vi "Fit Data.vi"(8 "error in":errorcluster, 10 "Data In":dbl[](array[numeric]), 11 "DFT-1 in":refnum<class "DFT-1.lvclass">) -> (0 "error out":errorcluster, 3 "DFT-1 out":refnum<class "DFT-1.lvclass">)   [LabVIEW 2014, in "Exponential Fit Library.lvlib" / "DFT-1.lvclass"]
doc: "Calculate tau from the first frequency component of the DFT using:\n\nbeta = 1/dt*ln(Re(F(k)/Im(F(k)*sin(w_k*dt) + cos(w_k*dt))\n\nwhere k = 1 and assuming unit spacing in time. Then, \n\ntau = 1/beta\n\nThe scale (A) and offset (B) are calculated as:\n\nA = (w^2+k^2)/ k*Re[F(n=1)]*dt/(1-exp(-k*tm)\nB = F(0)/N - A/(k*tm)*[1-exp(-k*tm)]\n\nwhere N is the number of samples, k = 1/tau, w = omega = 2*pi/tm, tm = N*dt, F(0) is the DC component of the FFT and Re[F(n=1)] is the real term of the first frequency component in the FFT spectrum. These computations are taken from Mazurenka et al. (2005) and are used in the determination of the uncertainty in the term tau (e_tau)."
uses:
  DFT-1.lvclass
  Fit Exponential.lvclass/Fit Exponential.ctl
  DFT-1.lvclass/DFT-1.ctl
  <vilib>/Analysis/2dsp.llb/Real FFT.vi
  Read Size.vi
  Read Sin.vi
  Read Cos.vi
  Read Dt.vi
  Write Output.vi
  Fit Exponential.lvclass
  <vilib>/Analysis/NI_AALPro.lvlib
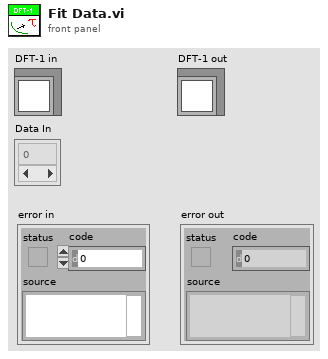
[diagram p1: front panel]
types:
  T1 = cluster{"A":dbl, "B":dbl, "tau":dbl, "e_tau":dbl}
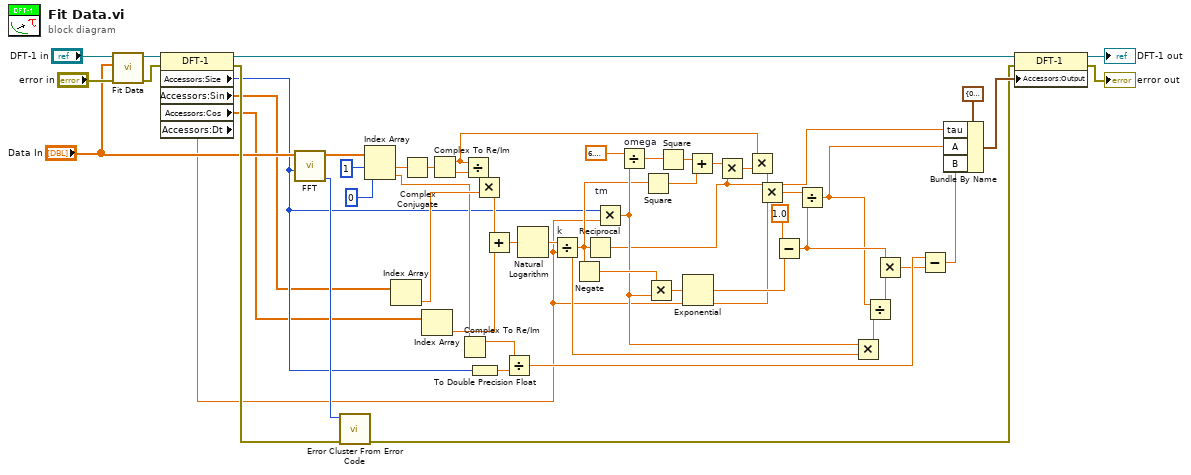
[diagram p0: block diagram]
diagram:
  n1 = call-parent "Fit Data.vi"("error in"="error in", "Data In"="Data In", "Fit Exponential in"="DFT-1 in") -> ("error out"=w16:errorcluster, "Fit Exponential out"=w17:refnum<class "DFT-1.lvclass">)  [unwired: 7 in]
  n2 = property class="DFT-1"(reference=w17, error in=w16) -> (reference out=w9:refnum<class "DFT-1.lvclass">, error out=w15:errorcluster, "Accessors:Size"=w13:i32, "Accessors:Sin"=w12:dbl[], "Accessors:Cos"=w11:dbl[], "Accessors:Dt"=w10:dbl)
  n3 = call-poly <vilib>:"FFT.vi"("FFT size"=w13, "X"="Data In") -> ("error"=w18:i32, "FFT {X}"=w46:cdb[])  [unwired: 1 in, 7 out]
  n4 = call <vilib>:"Error Cluster From Error Code.vi"("error in (no error)"=w15, "error code (0)"=w18) -> ("error out"=w3:errorcluster)  [unwired: 7 in]
  n5 = Index Array(array=w46, index #1=1 ("index"), index #2=0 ("index")) -> (element #1=w44:cdb, element #2=w20:cdb)
  n6 = Index Array(array=w12) -> (element=w48:dbl)  [unwired: 1 in]
  n7 = Complex Conjugate(1:w44) -> (0:w49:cdb)
  n8 = Index Array(array=w11) -> (element=w47:dbl)  [unwired: 1 in]
  n9 = Complex To Re/Im(x + iy=w49) -> (x=w37:dbl, y=w50:dbl)
  n10 = Complex To Re/Im(x + iy=w20) -> (x=w19:dbl)  [unwired: 1 out]
  n11 = Divide(x=w37, y=w50) -> (x/y=w53:dbl)
  n12 = To Double Precision Float(number=w13) -> (double precision float=w21:dbl)
  n13 = Multiply(x=w53, y=w48) -> (x*y=w52:dbl)
  n14 = Add(x=w52, y=w47) -> (x+y=w51:dbl)
  n15 = Divide(x=w19, y=w21) -> (x/y=w28:dbl)
  n16 = Natural Logarithm(1:w51) -> (0:w43:dbl)
  n17 = Divide "k"(x=w43, y=w10) -> (x/y=w22:dbl)
  n18 = Negate(x=w22) -> (-x=w33:dbl)
  n19 = Reciprocal(x=w22) -> (1/x=w1:dbl)
  n20 = Multiply "tm"(x=w13, y=w10) -> (x*y=w23:dbl)
  n21 = Divide "omega"(x=6.283185307179586, y=w23) -> (x/y=w41:dbl)
  n22 = Square(x=w22) -> (x^2=w40:dbl)
  n23 = Multiply(x=w33, y=w23) -> (x*y=w32:dbl)
  n24 = Square(x=w41) -> (x^2=w39:dbl)
  n25 = Exponential(1:w32) -> (0:w31:dbl)
  n26 = Add(x=w39, y=w40) -> (x+y=w38:dbl)
  n27 = Multiply(x=w38, y=w1) -> (x*y=w36:dbl)
  n28 = Multiply(x=w37, y=w36) -> (x*y=w35:dbl)
  n29 = Multiply(x=w35, y=w10) -> (x*y=w30:dbl)
  n30 = Subtract(x=1.0, y=w31) -> (x-y=w26:dbl)
  n31 = Divide ("A")(x=w30, y=w26) -> (x/y=w4:dbl)
  n32 = Multiply(x=w23, y=w22) -> (x*y=w27:dbl)
  n33 = Divide(x=w4, y=w27) -> (x/y=w25:dbl)
  n34 = Multiply(x=w26, y=w25) -> (x*y=w24:dbl)
  n35 = Subtract ("B")(x=w28, y=w24) -> (x-y=w5:dbl)
  n36 = Bundle By Name(cluster=T1 {"A"=0.0, "B"=0.0, "tau"=0.0, "e_tau"=0.0} ("Output"), "tau"=w1, "A"=w4, "B"=w5) -> (w6:T1)
  n37 = property class="DFT-1"(reference=w9, error in=w3, "Accessors:Output"=w6) -> (reference out=→"DFT-1 out":refnum<class "DFT-1.lvclass">, error out=→"error out":errorcluster)
